vi "Basic.vi"   [LabVIEW 2013]
uses:
  <vilib>/Rock Robotics/WPI/Solenoid/WPI_SolenoidValue.ctl
  Robot Global Data.vi
  <vilib>/Rock Robotics/WPI/Solenoid/WPI_SolenoidSetEnum.vi
types:
  T1 = typedef "WPI_SolenoidValue.ctl" = enum16{"Off", "On", "Forward", "Reverse"}
  T2 = enum16{"Manual Extend", "Manual Retract", "Shoot", "Wait"}
  T3 = typedef "WPI_SolenoidDevRef.ctl" = cluster{"DevStatus":errorcluster, "Solenoid Module":T4, "Forward Solenoid Channel":T5, "Reverse Solenoid Channel":T5}
  T4 = typedef "FPGA_TypedefSolenoidModule.ctl" = enum16{"Solenoid Module 1", "Solenoid Module 2"}
  T5 = typedef "WPI_SolenoidChannel.ctl" = enum8{"Solenoid 1", "Solenoid 2", "Solenoid 3", "Solenoid 4", "Solenoid 5", "Solenoid 6", "Solenoid 7", "Solenoid 8", "Invalid"}
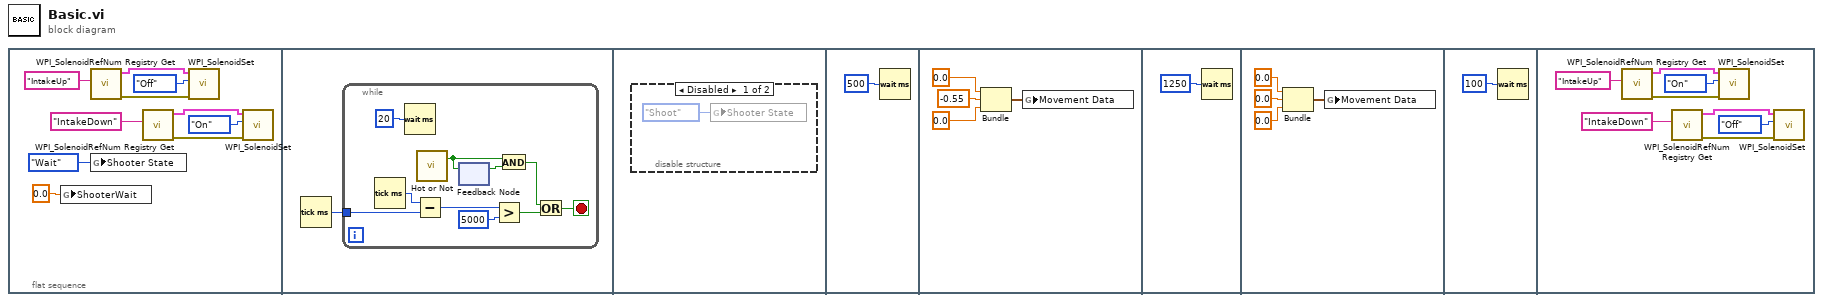
[diagram p0: block diagram]
diagram:
  n1 = flat-sequence {
    frame #0 {
      n2 = global write "Robot Global Data.vi" "ShooterWait"(0.0 ("ShooterWait")) -> ()
      n3 = call <vilib>:"WPI_SolenoidRefNum Registry Get.vi"("refnum name"="IntakeUp") -> ("error out"=w5:errorcluster, "SolenoidDevRef"=w6:T3)  [unwired: 9 in]
      n4 = global write "Robot Global Data.vi" "Shooter State"(T2."Wait" ("Shooter State")) -> ()
      n5 = call <vilib>:"WPI_SolenoidRefNum Registry Get.vi"("refnum name"="IntakeDown") -> ("error out"=w2:errorcluster, "SolenoidDevRef"=w3:T3)  [unwired: 9 in]
      n6 = call-poly <vilib>:"WPI_SolenoidSet.vi"("error in (no error)"=w5, "Value"=WPI_SolenoidValue."Off", "SolenoidDevRef"=w6) -> ()  [unwired: 7 in, 2 out]
      n7 = call-poly <vilib>:"WPI_SolenoidSet.vi"("error in (no error)"=w2, "Value"=WPI_SolenoidValue."On", "SolenoidDevRef"=w3) -> ()  [unwired: 7 in, 2 out]
    }
    frame #1 {
      n8 = Tick Count (ms)() -> (millisecond timer value=w11:u32)
      n9 = while {
        tunnel: w11 -> [w18]
        stop <- w21 stop-if-true
        n10 = Tick Count (ms)() -> (millisecond timer value=w19:u32)
        n11 = Wait (ms)(milliseconds to wait=u32 20) -> ()  [unwired: 1 out]
        n12 = Subtract(x=w19, y=w18) -> (x-y=w17:u32)
        n13 = call "Hot or Not.vi"() -> ("HotOrNot"=w13:bool)  [unwired: 4 in]
        n14 = feedback-in #1(w13) -> ()
        n15 = feedback #1() -> (w12:bool)  [unwired: 1 in]
        n16 = Greater?(x=w17, y=u32 5000) -> (0:w15:bool)
        n17 = And(x=w13, y=w12) -> (x .and. y?=w14:bool)
        n18 = Or(x=w14, y=w15) -> (x .or. y?=w21:bool)
      }
    }
    frame #2 {
      n19 = disable-structure shown="Disabled" {
        frame Disabled {
          n20 = global write "Robot Global Data.vi" "Shooter State"(T2."Shoot" ("Shooter State")) -> ()
        }
        frame Enabled {
        }
      }
    }
    frame #3 {
      n21 = Wait (ms)(milliseconds to wait=u32 500) -> ()  [unwired: 1 out]
    }
    frame #4 {
      n22 = Bundle(0.0, -0.55, 0.0) -> (w24:cluster{dbl, dbl, dbl})  [unwired: 1 in]
      n23 = global write "Robot Global Data.vi" "Movement Data"(w24) -> ()
    }
    frame #5 {
      n24 = Wait (ms)(milliseconds to wait=u32 1250) -> ()  [unwired: 1 out]
    }
    frame #6 {
      n25 = Bundle(0.0, 0.0, 0.0) -> (w29:cluster{dbl, dbl, dbl})  [unwired: 1 in]
      n26 = global write "Robot Global Data.vi" "Movement Data"(w29) -> ()
    }
    frame #7 {
      n27 = Wait (ms)(milliseconds to wait=u32 100) -> ()  [unwired: 1 out]
    }
    frame #8 {
      n28 = call <vilib>:"WPI_SolenoidRefNum Registry Get.vi"("refnum name"="IntakeUp") -> ("error out"=w37:errorcluster, "SolenoidDevRef"=w38:T3)  [unwired: 9 in]
      n29 = call <vilib>:"WPI_SolenoidRefNum Registry Get.vi"("refnum name"="IntakeDown") -> ("error out"=w34:errorcluster, "SolenoidDevRef"=w35:T3)  [unwired: 9 in]
      n30 = call-poly <vilib>:"WPI_SolenoidSet.vi"("error in (no error)"=w37, "Value"=WPI_SolenoidValue."On", "SolenoidDevRef"=w38) -> ()  [unwired: 7 in, 2 out]
      n31 = call-poly <vilib>:"WPI_SolenoidSet.vi"("error in (no error)"=w34, "Value"=WPI_SolenoidValue."Off", "SolenoidDevRef"=w35) -> ()  [unwired: 7 in, 2 out]
    }
  }
